vi "Write ADU Packet.vi"(8 "error in (no error)":errorcluster, 9 "Modbus data unit":refnum<class "Modbus Data Unit (PDU).lvclass">, 10 "protocol layer":refnum<class "Network Protocol.lvclass">, 11 "transmission data unit in":refnum<class "Transmission Data Unit.lvclass">) -> (0 "error out":errorcluster, 2 "protocol layer out":refnum<class "Network Protocol.lvclass">, 3 "transmission data unit out":refnum<class "Transmission Data Unit.lvclass">)   [LabVIEW 2020, in "SubVIs.lvlib" / "Transmission Data Unit.lvclass"]
doc: "This method accepts a modbus modbus data unit as input and writes the data of the PDU onto the selected network."
uses:
  <vilib>/Modbus/subvis/Transmission Data Unit (ADU)/Transmission Data Unit/Transmission Data Unit.lvclass
  <vilib>/Modbus/subvis/Modbus Data Unit (PDU)/Modbus Data Unit (PDU).lvclass
  <vilib>/Modbus/subvis/Protocol/Interfaces/Network Protocol/Network Protocol.lvclass
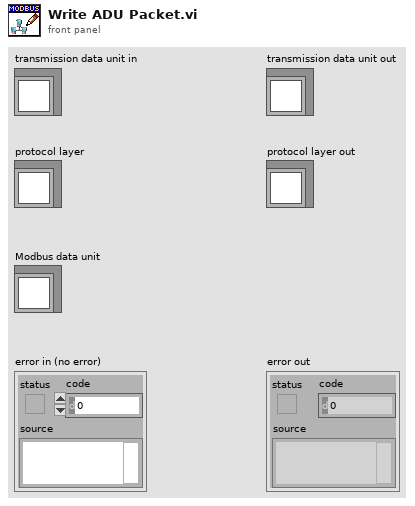
[diagram p1: front panel]
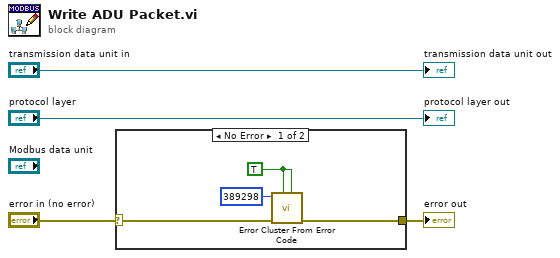
[diagram p0: block diagram]
diagram:
  n1 = case shown="No Error" "error in (no error)" {
    selector: "error in (no error)" -> [w7 w9]
    tunnel: [w8 w9] -> w1
    frame No Error {
      w5 = TRUE ("show call chain? (False)")
      n2 = call <vilib>:"Error Cluster From Error Code.vi"("is warning? (False)"=w5, "show call chain? (False)"=w5, "error in (no error)"=w7, "error code (0)"=389298) -> ("error out"=w8:errorcluster)  [unwired: 5 in]
    }
    frame Error {
    }
  }
  "error out" <- w1
  "transmission data unit out" <- "transmission data unit in"
  "protocol layer out" <- "protocol layer"
